vi "Fire Bullet.vi"(8 "error in (no error)":errorcluster, 10 "buttons":bool[](array[boolean]), 11 "Game Data in":T1) -> (0 "error out":errorcluster, 3 "Game Data out":T1)   [LabVIEW 2025]
uses:
  Game Data.ctl
  Bullet Data.ctl
  Game State.ctl
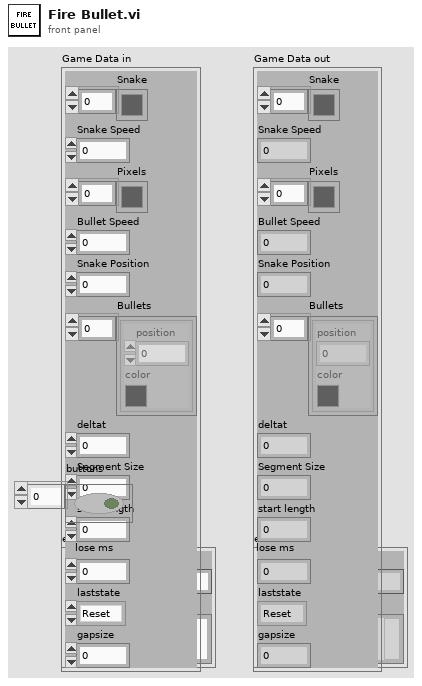
[diagram p1: front panel]
types:
  T1 = typedef "Game Data.ctl" = cluster{"Snake":u32[], "Snake Speed":dbl, "Pixels":u32[], "Bullet Speed":dbl, "Snake Position":dbl, "Bullets":T2[], "deltat":dbl, "Segment Size":dbl, "start length":u32, "lose ms":u32, "laststate":T3, "gapsize":i32}
  T2 = typedef "Bullet Data.ctl" = cluster{"position":dbl, "color":u32}
  T3 = typedef "Game State.ctl" = enum16{"Reset", "Idle", "Start", "Playing", "Win", "Lose"}
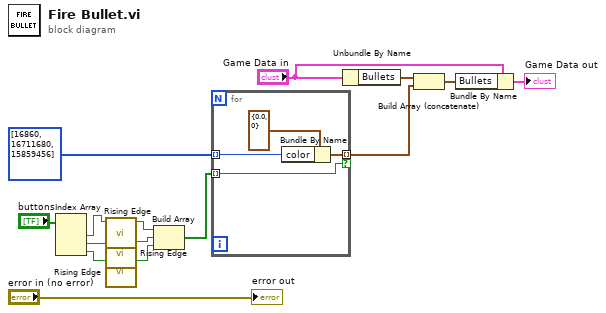
[diagram p0: block diagram]
diagram:
  n1 = Index Array(array="buttons") -> (element #1=w4:bool, element #2=w3:bool, element #3=w2:bool)  [unwired: 3 in]
  n2 = call "Rising Edge.vi"("signal"=w4) -> ("edge?"=w8:bool)  [unwired: 10 in]
  n3 = call "Rising Edge.vi"("signal"=w3) -> ("edge?"=w7:bool)  [unwired: 10 in]
  n4 = call "Rising Edge.vi"("signal"=w2) -> ("edge?"=w6:bool)  [unwired: 10 in]
  n5 = Build Array(w8, w7, w6) -> (w1:bool[])
  n6 = for {
    tunnel: [w18] -> w9 mode=indexing if=w16
    tunnel: u32[] [16860, 16711680, 15859456] -> [w17] mode=indexing
    tunnel: w1 -> [w16] mode=indexing
    n7 = Bundle By Name(cluster=T2 {"position"=0.0, "color"=0} ("Bullet"), "color"=w17) -> (w18:T2)
  }
  n8 = Unbundle By Name("Game Data in") -> ("Bullets"=w11:T2[])
  n9 = Build Array (concatenate)(w11, w9) -> (w10:T2[])
  n10 = Bundle By Name(cluster="Game Data in", "Bullets"=w10) -> (→"Game Data out":T1)
  "error out" <- "error in (no error)"
